vi "Read Transfer speed.vi"(8 "error in (no error)":errorcluster, 11 "ScopeBase in":refnum<class "ScopeBase.lvclass">) -> (0 "error out":errorcluster, 2 "Tranfer speed":T1, 3 "ScopeBase out":refnum<class "ScopeBase.lvclass">)   [LabVIEW 2018, in "ScopeBase.lvclass"]
uses:
  ScopeBase.lvclass
  controls/host_transfer_speed.ctl
  ScopeBase.lvclass/ScopeBase.ctl
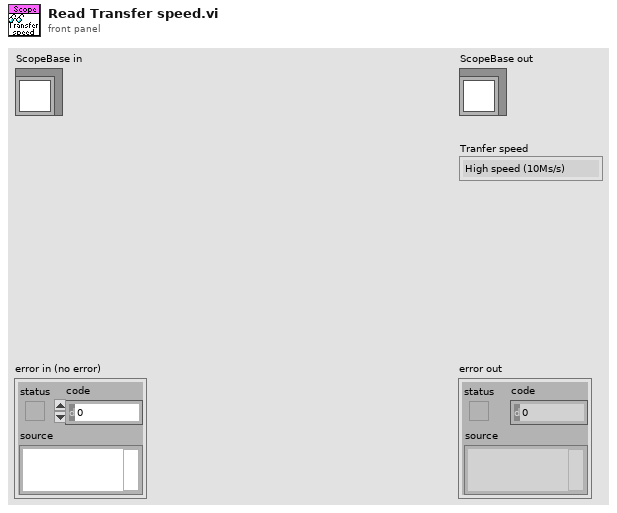
[diagram p1: front panel]
types:
  T1 = typedef "host_transfer_speed.ctl" = enum16{"High speed (10Ms/s)", "Low speed (1Ms/s)", "Ultra low speed (50kS/s)"}
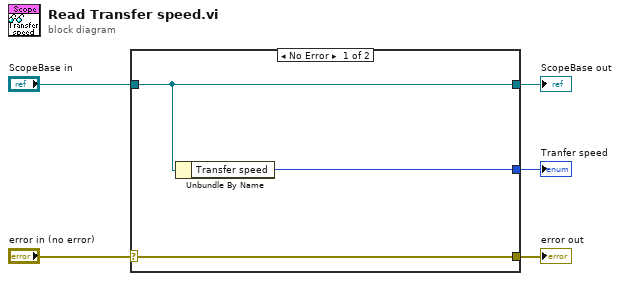
[diagram p0: block diagram]
diagram:
  n1 = case shown="No Error" "error in (no error)" {
    selector: "error in (no error)" -> [w8 w9]
    tunnel: [w8 w9] -> w4
    tunnel: [w7 w10] -> w2
    tunnel: "ScopeBase in" -> [w7 w10]
    tunnel: [w6 _] -> w1
    frame No Error {
      n2 = Unbundle By Name(w7) -> ("Transfer speed"=w6:T1)
    }
    frame Error {
    }
  }
  "error out" <- w4
  "ScopeBase out" <- w2
  "Tranfer speed" <- w1
